vi "kalman_test_2.vi"() -> ()   [LabVIEW 2016]
uses:
  <vilib>/Analysis/Matrix/Datatypes/RealMatrix.ctl
  <vilib>/Analysis/Matrix/NI_Matrix.lvlib
panel:
  out "Waveform Chart":T1(graph)
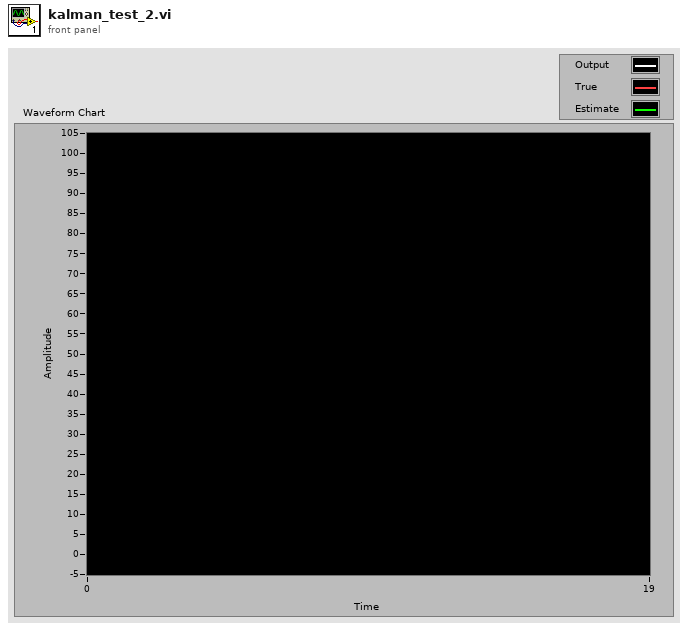
[diagram p1: front panel]
types:
  T1 = cluster{"Real Matrix Element":dbl, "Real Matrix Element":dbl, "Real Matrix Element":dbl}
  T2 = cluster{"Real Matrix Element":dbl, "Real Matrix Element":dbl, "Real Matrix Element":dbl}[]
  T3 = typedef "NI_Matrix.lvlib/RealMatrix.ctl" = dbl[][]
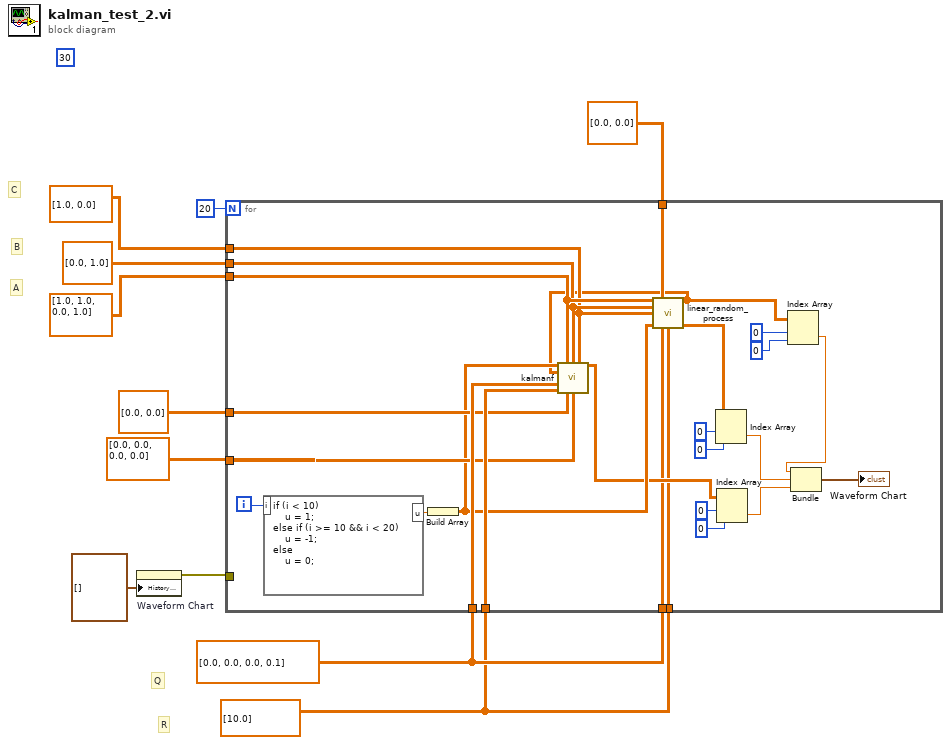
[diagram p0: block diagram]
diagram:
  w1 = T3 [[10.0]] ("Q")
  w2 = T3 [[0.0, 0.0], [0.0, 0.1]] ("Q")
  (unwired) 30
  # "C"
  # "B"
  # "A"
  # "R"
  # "Q"
  n1 = property on="Waveform Chart" class="WFChart (strict)"("History Data"=T2 []) -> (error out=w4:errorcluster)  [unwired: 2 in, 1 out]
  n2 = for {
    N: 20 -> [_]
    tunnel: T3 [[1.0, 1.0], [0.0, 1.0]] ("A") -> [w37]
    tunnel: T3 [[0.0], [1.0]] ("B") -> [w36]
    tunnel: T3 [[1.0, 0.0]] ("xhat") -> [w35]
    tunnel: w2 -> [w34]
    tunnel: w1 -> [w33]
    tunnel: T3 [[0.0], [0.0]] ("B") -> [w32]
    tunnel: w1 -> [w12]
    tunnel: w2 -> [w13]
    tunnel: T3 [[0.0], [0.0]] ("B") -> [w31]
    tunnel: T3 [[0.0, 0.0], [0.0, 0.0]] ("B") -> [w30]
    tunnel: w4 -> [_]
    i -> [w29]
    n3 = formula code="if (i < 10)\n    u = 1;\nelse if (i >= 10 && i < 20)\n    u = -1;\nelse \n    u = 0;"("i"=w29) -> ("u"=w28:dbl)
    n4 = Build Array(w28) -> (w27:T3)
    n5 = call "linear_random_process.vi"("A"=w37, "x0"=w32, "B"=w36, "C"=w35, "u"=w27, "Q"=w13, "R"=w12) -> ("y"=w14:T3, "x"=w24:T3)  [unwired: 7 in]
    n6 = call "kalmanf.vi"("u"=w27, "A"=w37, "B"=w36, "C"=w35, "y"=w14, "Q"=w34, "R"=w33, "xhat0"=w31, "P0"=w30) -> ("xhat"=w21:T3)  [unwired: 6 in]
    n7 = Index Array(array=w24, index (row)=0, index (col)=0) -> (element=w20:dbl)
    n8 = Index Array(array=w21, index (row)=0, index (col)=0) -> (element=w19:dbl)
    n9 = Index Array(array=w14, index (row)=0, index (col)=0) -> (element=w15:dbl)
    n10 = Bundle("Real Matrix Element"=w15, "Real Matrix Element"=w20, "Real Matrix Element"=w19) -> (→"Waveform Chart":T1)  [unwired: 1 in]
  }
